vi "Rinse_syringe_subVI_BM.vi"(4 "COM Port":refnum<visa-resource-name>="COM12", 7 "Pump Parameters":T1={"Speed 1"="150", "Speed 2"="250", "Speed 3"="450", "Speed 4"="250", "UW/Sample"="5", "Sparge"="2", "Std"="4", "Waste"="15", "Air"="14", "Milli-Q"="1", "H2SO4"="6", "NaOH"="3", "Catalyst"="7", "Cell (H+ side)"="8", "Cell (sample side)"="9", "NaCl"="11"}, 8 "N syringe rinses":i32=3, 9 "step to ml":dbl=1920.0) -> ()   [LabVIEW 2021]
panel:
  out "Full Command":string="V450O1P38400O15D38400"
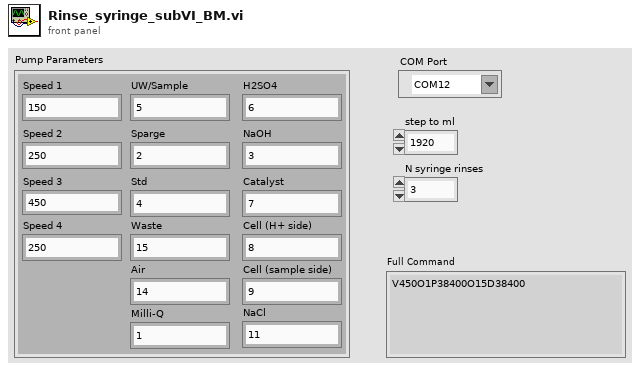
[diagram p1: front panel]
types:
  T1 = cluster{"Speed 1":string, "Speed 2":string, "Speed 3":string, "Speed 4":string, "UW/Sample":string, "Sparge":string, "Std":string, "Waste":string, "Air":string, "Milli-Q":string, "H2SO4":string, "NaOH":string, "Catalyst":string, "Cell (H+ side)":string, "Cell (sample side)":string, "NaCl":string}
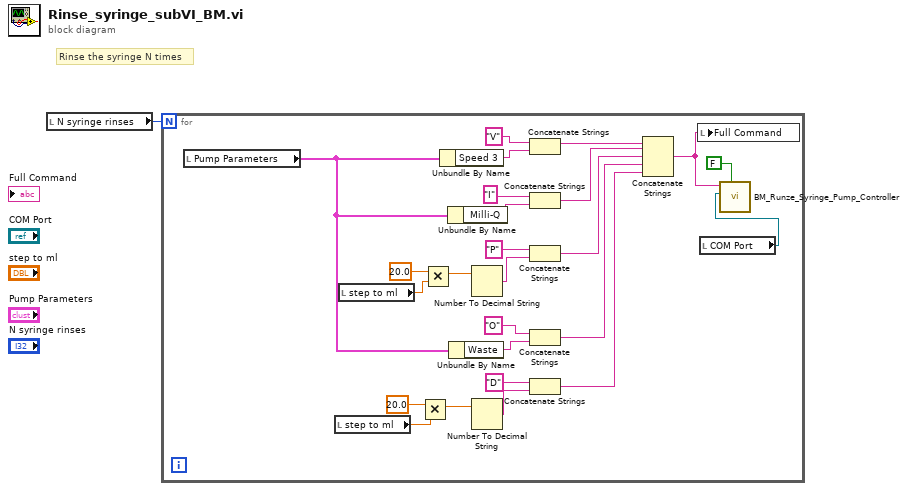
[diagram p0: block diagram]
diagram:
  # "Rinse the syringe N times"
  n1 = local read "N syringe rinses"() -> (w1:i32)
  n2 = for {
    N: w1 -> [_]
    n3 = local read "Pump Parameters"() -> (w8:T1)
    n4 = local read "step to ml"() -> (w9:dbl)
    n5 = local read "step to ml"() -> (w20:dbl)
    n6 = Multiply(x=20.0, y=w9) -> (x*y=w12:dbl)
    n7 = Multiply(x=20.0, y=w20) -> (x*y=w21:dbl)
    n8 = Unbundle By Name(w8) -> ("Speed 3"=w16:string)
    n9 = Unbundle By Name(w8) -> ("Milli-Q"=w23:string)
    n10 = Unbundle By Name(w8) -> ("Waste"=w14:string)
    n11 = Number To Decimal String(number=w21) -> (decimal integer string=w18:string)  [unwired: 1 out]
    n12 = Number To Decimal String(number=w12) -> (decimal integer string=w11:string)  [unwired: 1 out]
    n13 = Concatenate Strings("V", w16) -> (w7:string)
    n14 = Concatenate Strings("I", w23) -> (w6:string)
    n15 = Concatenate Strings("P" ("string"), w18) -> (w5:string)
    n16 = Concatenate Strings("O", w14) -> (w4:string)
    n17 = Concatenate Strings("D" ("string"), w11) -> (w3:string)
    n18 = Concatenate Strings(w7, w6, w5, w4, w3) -> (w24:string)
    n19 = local write "Full Command"(w24) -> ()
    n20 = local read "COM Port"() -> (w25:refnum<visa-resource-name>)
    n21 = call "BM_Runze_Syringe_Pump_Controller.vi"("Initialize Plunger?"=FALSE ("Initialize?"), "COM Port (Runze)"=w25, "Enter Command"=w24) -> ()  [unwired: 6 in, 3 out]
  }
